vi "Read States.vi"(8 "error in (no error)":errorcluster, 11 "WaitPassTactic in":refnum<class "WaitPassTactic.lvclass">) -> (0 "error out":errorcluster, 2 "States":enum16{"State 0", "State 1", "State 2", "Exit"}(ring), 3 "WaitPassTactic out":refnum<class "WaitPassTactic.lvclass">)   [LabVIEW 2024, in "WaitPassTactic.lvclass"]
uses:
  WaitPassTactic.lvclass
  WaitPassTactic.lvclass/WaitPassTactic.ctl
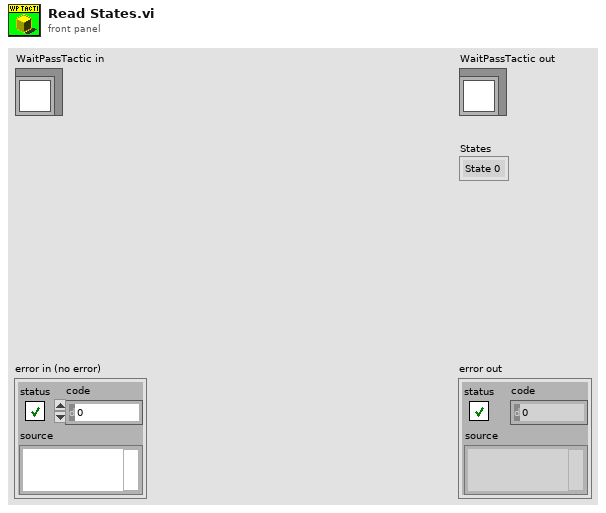
[diagram p1: front panel]
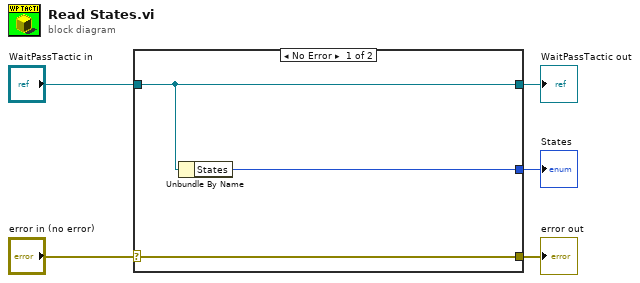
[diagram p0: block diagram]
diagram:
  n1 = case shown="No Error" "error in (no error)" {
    selector: "error in (no error)" -> [w8 w9]
    tunnel: [w8 w9] -> w4
    tunnel: [w7 w10] -> w2
    tunnel: "WaitPassTactic in" -> [w7 w10]
    tunnel: [w6 _] -> w1
    frame No Error {
      n2 = Unbundle By Name(w7) -> ("States"=w6:enum16{"State 0", "State 1", "State 2", "Exit"})
    }
    frame Error {
    }
  }
  "error out" <- w4
  "WaitPassTactic out" <- w2
  "States" <- w1
